vi "AH2500_Splitt_Cluster.vi"(0 "AH2500-Cluster":T3={"Capacity Graphic"=[], "Loss Graphic"=[], "Update AH2500"=FALSE, "Capacity"=0.0, "Loss"=0.0, "AVerage"=enum."5", "ALternate"=enum."1", "BIas"=enum."Disabled", "V excitation"=enum."15.00"}) -> (1 "AH2500-Control":T2, 2 "AH2500-Status":T1)   [LabVIEW 2019]
uses:
  AH2500/AH2500-Cluster.ctl
  AH2500/AH2500-Control.ctl
  AH2500/AH2500-Status.ctl
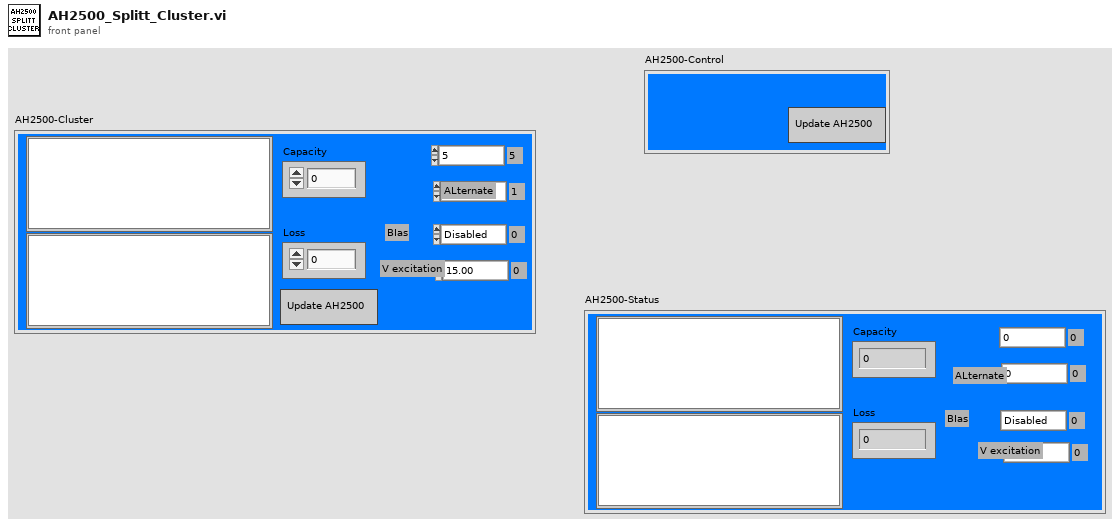
[diagram p1: front panel]
types:
  T1 = typedef "AH2500-Status.ctl" = cluster{"Capacity Graphic":dbl[][], "Loss Graphic":dbl[][], "Capacity":dbl, "Loss":dbl, "AVerage":enum16{"0", "1", "2", "3", "4", "5", "6", "7", "8", "9", "10", "11", "12", "13", "14", "15"}, "ALternate":enum16{"0", "1", "2", "3", "4", "5", "6", "7"}, "BIas":enum16{"Disabled", "100 MOhm", "1 MOhm"}, "V excitation":enum16{"15.00", "7.50", "3.75", "3.00", "1.50", "0.750", "0.375", "0.250", "0.125", "0.100", "0.050", "0.030", "0.015", "0.010", "0.0050", "0.0030", "0.0015", "0.0010", "0.0005"}}
  T2 = typedef "AH2500-Control.ctl" = cluster{"Update AH2500":bool}
  T3 = typedef "AH2500-Cluster.ctl" = cluster{"Capacity Graphic":dbl[][], "Loss Graphic":dbl[][], "Update AH2500":bool, "Capacity":dbl, "Loss":dbl, "AVerage":enum16{"0", "1", "2", "3", "4", "5", "6", "7", "8", "9", "10", "11", "12", "13", "14", "15"}, "ALternate":enum16{"0", "1", "2", "3", "4", "5", "6", "7"}, "BIas":enum16{"Disabled", "100 MOhm", "1 MOhm"}, "V excitation":enum16{"15.00", "7.50", "3.75", "3.00", "1.50", "0.750", "0.375", "0.250", "0.125", "0.100", "0.050", "0.030", "0.015", "0.010", "0.0050", "0.0030", "0.0015", "0.0010", "0.0005"}}
  T4 = enum16{"0", "1", "2", "3", "4", "5", "6", "7", "8", "9", "10", "11", "12", "13", "14", "15"}
  T5 = enum16{"15.00", "7.50", "3.75", "3.00", "1.50", "0.750", "0.375", "0.250", "0.125", "0.100", "0.050", "0.030", "0.015", "0.010", "0.0050", "0.0030", "0.0015", "0.0010", "0.0005"}
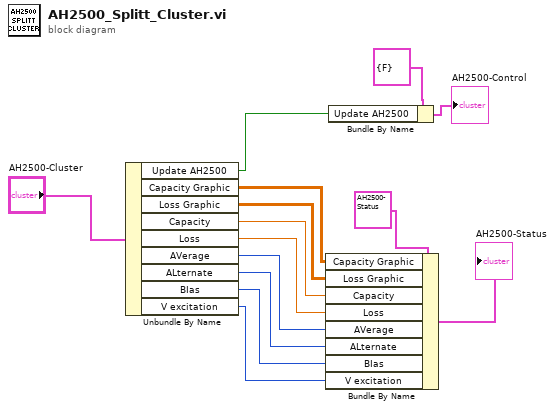
[diagram p0: block diagram]
diagram:
  n1 = Unbundle By Name("AH2500-Cluster") -> ("Update AH2500"=w9:bool, "Capacity Graphic"=w8:dbl[][], "Loss Graphic"=w7:dbl[][], "Capacity"=w6:dbl, "Loss"=w5:dbl, "AVerage"=w4:T4, "ALternate"=w3:enum16{"0", "1", "2", "3", "4", "5", "6", "7"}, "BIas"=w2:enum16{"Disabled", "100 MOhm", "1 MOhm"}, "V excitation"=w1:T5)
  n2 = Bundle By Name(cluster=T1 {"Capacity Graphic"=[], "Loss Graphic"=[], "Capacity"=0.0, "Loss"=0.0, "AVerage"=enum."0", "ALternate"=enum."0", "BIas"=enum."Disabled", "V excitation"=enum."15.00"} ("AH2500-Status"), "Capacity Graphic"=w8, "Loss Graphic"=w7, "Capacity"=w6, "Loss"=w5, "AVerage"=w4, "ALternate"=w3, "BIas"=w2, "V excitation"=w1) -> (→"AH2500-Status":T1)
  n3 = Bundle By Name(cluster=T2 {"Update AH2500"=FALSE} ("AH2500-Control"), "Update AH2500"=w9) -> (→"AH2500-Control":T2)
